vi "OAuth.vi"() -> ()   [LabVIEW 2016]
panel:
  in  "File Names":string[](array[string])=["Asana_Authorization_Code.txt", "Asana_Access_Token.txt", "Asana_Refresh_Token.txt"]
  out "Codes":T1
  out "Auth Time Out":dbl
  out "error out":errorcluster
  in  "Auth Time In":dbl
  in  "error in (no error)":errorcluster
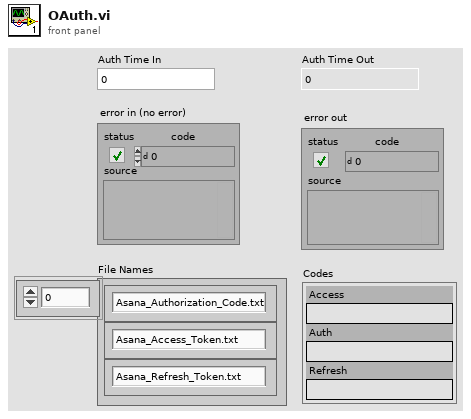
[diagram p1: front panel]
types:
  T1 = cluster{"Access":string, "Auth":string, "Refresh":string}
  T2 = cluster{"Auth Code":path, "Access Token":path, "Refresh Token":path}
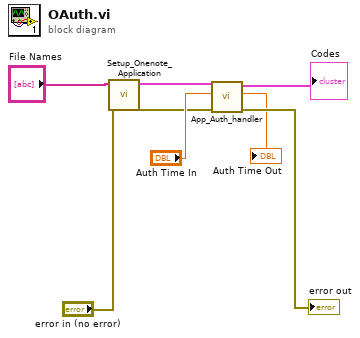
[diagram p0: block diagram]
diagram:
  n1 = call "Setup_Onenote_Application.vi"("error in (no error)"="error in (no error)", "Array"="File Names") -> ("error out"=w4:errorcluster, "Paths"=w1:T2)  [unwired: 8 in]
  n2 = call "App_Auth_handler.vi"("error in (no error)"=w4, "Auth Time In"="Auth Time In", "Paths"=w1) -> ("error out"=→"error out":errorcluster, "Auth Time Out"=→"Auth Time Out":dbl, "Codes"=→"Codes":T1)  [unwired: 6 in]
